vi "Test_Copy_Pixmap_to_Image_ARGB.vi"(8 "error in (no error)":errorcluster, 11 "Test Case In":refnum<class "Image.lvclass">) -> (0 "error out":errorcluster, 3 "Test Case Out":refnum<class "Image.lvclass">)   [LabVIEW 2020]
uses:
  Image.lvclass
  C:/Program Files (x86)/National Instruments/LabVIEW 2020/vi.lib/Astemes/LUnit/Test Case.lvclass
  g_ar_toolkit.common/Image Size (Integer).ctl
  <vilib>/Astemes/LUnit/Test Case.lvclass/Test Case.ctl
  g_ar_toolkit.image/CreateEmptyImageARGB.vi
  g_ar_toolkit.image/CopyPixmapToImageIgnoreMaskARGB.vi
  4993e8ee-a06a-463a-9684-69129f64d5ce.vi
  g_ar_toolkit.image/CreateEmptyImageARGB.vi/3321fa97-f432-4e1e-8db9-a0df79aed21b.vi
  g_ar_toolkit.image/CopyPixmapToImageIgnoreMaskARGB.vi/80b1166a-8c06-443b-b271-eb6a715622f7.vi
  <vilib>/Astemes/LUnit/Append Pass Result.vi
  <vilib>/Astemes/LUnit/Append Fail Result.vi
  <vilib>/Astemes/LUnit/Describe Comparison.vi
  <vilib>/Astemes/LUnit/Compare Variants.vi
  g_ar_toolkit.image/FixPixmapColourArraySize.vi
  <vilib>/Astemes/LUnit/Variant to string.vi
  g_ar_toolkit.image/Default8bitColourMap.vi
  g_ar_toolkit.image/ARGBColourToU32.vi
  <vilib>/Utility/error.llb/Error Cluster From Error Code.vi
  <vilib>/picture/picture.llb/Draw Rectangle.vi
  <vilib>/picture/pictutil.llb/Picture to Pixmap.vi
  <vilib>/Utility/Data Type/Get Type Information.vi
  <vilib>/Utility/LVClass/Get LV Class Name.vi
  g_ar_toolkit.image/g_ar_toolkit.image.lvlib
  g_ar_toolkit.common/g_ar_toolkit.common.lvlib
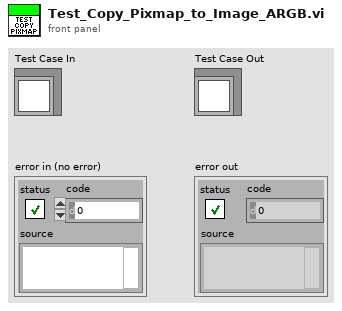
[diagram p1: front panel]
types:
  T1 = typedef "g_ar_toolkit.common.lvlib/Image Size (Integer).ctl" = cluster{"Width":u16, "Height":u16}
  T2 = typedef "imagedata.ctl" = cluster{"image type":i32, "image depth":i32, "image":u8[], "mask":u8[], "colors":u32[], "Rectangle":cluster{"left":i16, "top":i16, "right":i16, "bottom":i16}}
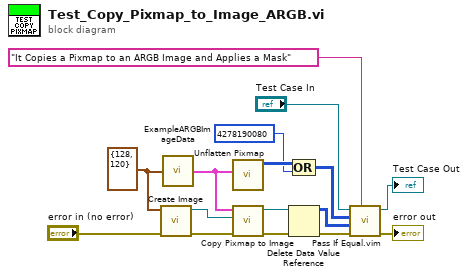
[diagram p0: block diagram]
diagram:
  w1 = T1 {"Width"=128, "Height"=120} ("Preallocated Image Size (Default - 0,0)")
  n1 = call-poly "Create Image.vi"("error in (no error)"="error in (no error)", "Preallocated Image Size (Default: 0,0)"=w1) -> ("error out"=w10:errorcluster, "New ARGB Image"=w9:refnum<data-value>)  [unwired: 8 in]
  n2 = call "ExampleARGBImageData.vi"("Image Size"=w1) -> ("RGB Image Data"=w5:T2)
  n3 = call <vilib>:"Unflatten Pixmap.vi"("image data"=w5) -> ("24-bit pixmap"=w4:u32[][])  [unwired: 4 in, 6 out]
  n4 = call-poly "Copy Pixmap to Image.vi"("error in (no error)"=w10, "ARGB Image Destination"=w9, "Pixmap Image Data"=w5) -> ("error out"=w8:errorcluster, "ARGB Image Destination (duplicate)"=w6:refnum<data-value>)  [unwired: 7 in]
  n5 = Delete Data Value Reference(data value reference=w6, error in=w8) -> (data value=w7:u32[][], error out=w11:errorcluster)
  n6 = Compound Arithmetic op=OR(w4, u32 4278190080) -> (w3:u32[][])
  n7 = call "Pass If Equal.vim"("Description"="It Copies a Pixmap to an ARGB Image and Applies a Mask", "error in (no error)"=w11, "Actual"=w7, "Expected"=w3, "LUnit Test Case In"="Test Case In") -> ("error out"=→"error out":errorcluster, "LUnit Test Case Out"=→"Test Case Out":refnum<class "Image.lvclass">)  [unwired: 5 in]
